vi "Connect.vi"(8 "error in (no error)":errorcluster, 11 "host":string) -> (0 "error out":errorcluster, 3 "handle":u64)   [LabVIEW 2015, in "ReDeX.lvlib"]
doc: "redex_lv_result redex_lv_connect(const char *host, redex_lv_handle *handle);"
uses:
  ReDeX.lvlib
  C:/ReDeX/ReDeX.dll
panel:
  out "function return":u32(ring)
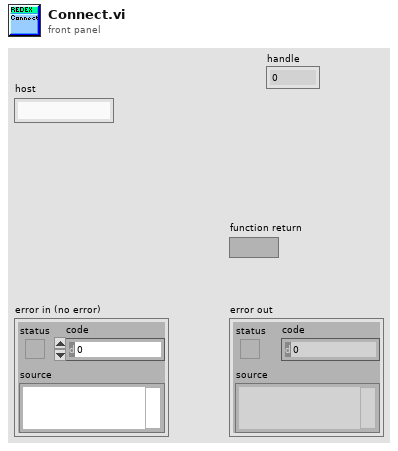
[diagram p1: front panel]
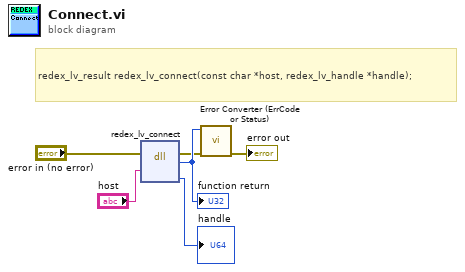
[diagram p0: block diagram]
diagram:
  # "redex_lv_result redex_lv_connect(const char *host, redex_lv_handle *handle);"
  n1 = dll-call lib="C:/ReDeX/ReDeX.dll" fn="redex_lv_connect"(error in="error in (no error)", "host"="host") -> (error out=w3:errorcluster, "return type"=w6:u32, "handle"=→"handle":u64)  [unwired: 4 in, 1 out]
  "function return" <- w6
  n2 = call "Error Converter (ErrCode or Status).vi"("error in (no error)"=w3, "error code"=w6) -> ("error out"=→"error out":errorcluster)  [unwired: 9 in]
